vi "Add Channel.vi"(7 "Highlight? (F)":bool, 8 "error in":errorcluster, 9 "Channel":T1, 10 "Name":string, 11 "Frame Ref":T3 format="%.0x") -> (0 "error out":errorcluster, 3 "Channel Ref out":T3 format="%.0x")   [LabVIEW 2020, in "Communication Bus Template Scripting.lvlib"]
uses:
  Communication Bus Template Scripting.lvlib
  <vilib>/NI VeriStand/Custom Device API/Custom Device Item Ref.ctl
  <vilib>/NI VeriStand/Custom Device API/Custom Device Channel.ctl
  <vilib>/NI VeriStand/Custom Device API/Custom Device Channel Type.ctl
  System Explorer/Constants.vi
  <vilib>/NI VeriStand/Custom Device API/Custom Device API.lvlib
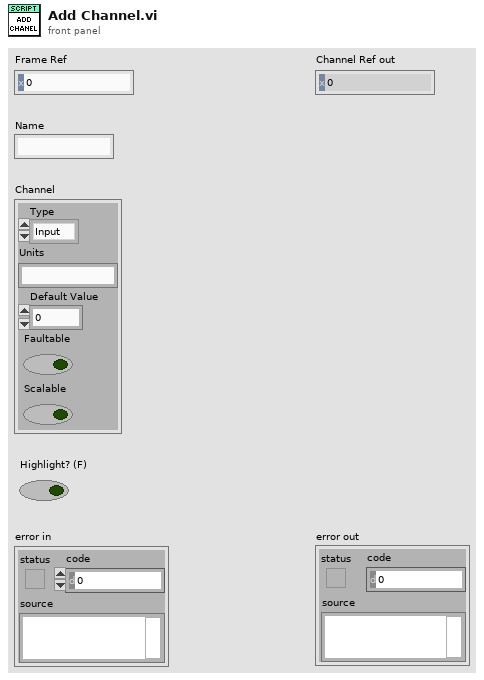
[diagram p1: front panel]
types:
  T1 = typedef "Custom Device API.lvlib/Custom Device Channel.ctl" = cluster{"Type":T2, "Units":string, "Default Value":dbl, "Faultable":bool, "Scalable":bool}
  T2 = typedef "Custom Device API.lvlib/Custom Device Channel Type.ctl" = enum16{"Input", "Output"}
  T3 = typedef "Custom Device API.lvlib/Custom Device Item Ref.ctl" = u64
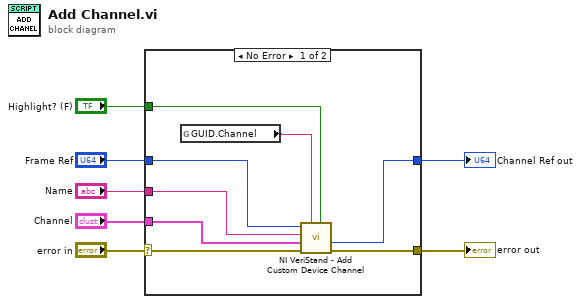
[diagram p0: block diagram]
diagram:
  n1 = case shown="No Error" "error in" {
    selector: "error in" -> [w15 w16]
    tunnel: [w14 w16] -> w6
    tunnel: "Frame Ref" -> [w12 _]
    tunnel: [w11 _] -> w4
    tunnel: "Name" -> [w13 _]
    tunnel: "Channel" -> [w10 _]
    tunnel: "Highlight? (F)" -> [w9 _]
    frame No Error {
      n2 = global read "Constants.vi" "GUID.Channel"() -> (w8:string)
      n3 = call <vilib>:"NI VeriStand - Add Custom Device Channel.vi"("Highlight? (F)"=w9, "GUID (Default Channel)"=w8, "error in (no error)"=w15, "Channel"=w10, "Channel Name"=w13, "Parent Ref in"=w12) -> ("error out"=w14:errorcluster, "Channel Ref"=w11:T3)  [unwired: 2 in, 2 out]
    }
    frame Error {
    }
  }
  "Channel Ref out" <- w4
  "error out" <- w6
